vi "总磷氨氮公式读取.vi"(8 "error in (no error)":errorcluster caption="错误输入（无错误）", 9 "量程":enum16{"低量程", "高量程"}(ring), 10 "测量模式":enum16{"水样测量", "空白核查", "跨度核查", "标样核查", "加标回收"}(ring), 11 "测量参数":enum16{"氨氮", "总磷"}(ring)) -> (0 "error out":errorcluster caption="错误输出", 3 "公式":cluster{"X^2":dbl, "X":dbl, "b":dbl})   [LabVIEW 2016, in "氨氮.lvlib"]
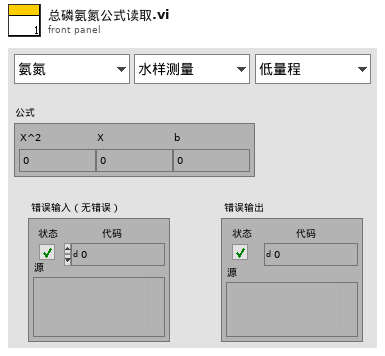
[diagram p1: front panel]
types:
  T1 = cluster{"FLOAT[0]":sgl, "FLOAT[1]":sgl, "FLOAT[2]":sgl}
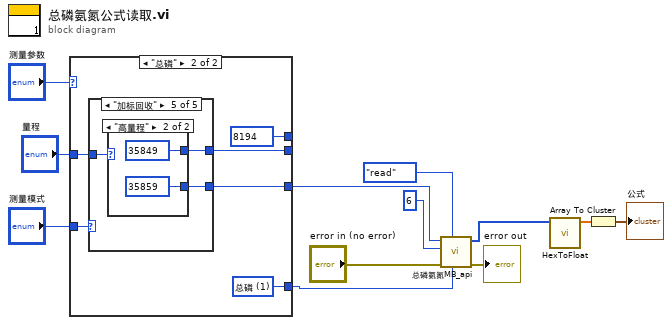
[diagram p0: block diagram]
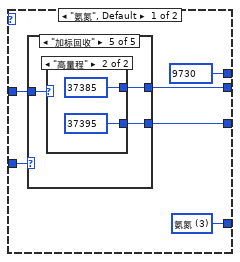
[diagram p2: hidden frame]
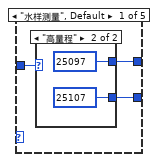
[diagram p3: hidden frame]
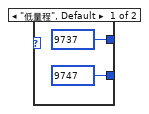
[diagram p4: hidden frame]
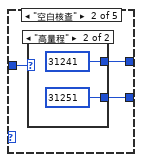
[diagram p5: hidden frame]
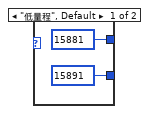
[diagram p6: hidden frame]
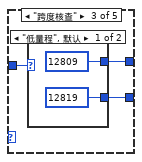
[diagram p7: hidden frame]
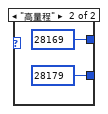
[diagram p8: hidden frame]
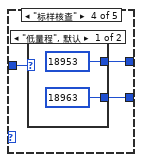
[diagram p9: hidden frame]
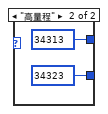
[diagram p10: hidden frame]
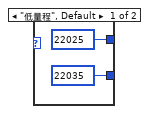
[diagram p11: hidden frame]
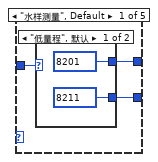
[diagram p12: hidden frame]
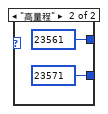
[diagram p13: hidden frame]
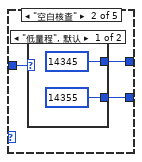
[diagram p14: hidden frame]
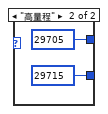
[diagram p15: hidden frame]
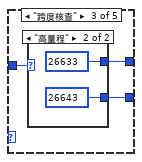
[diagram p16: hidden frame]
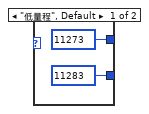
[diagram p17: hidden frame]
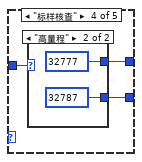
[diagram p18: hidden frame]
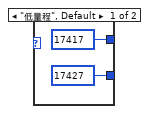
[diagram p19: hidden frame]
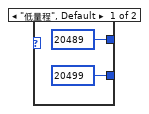
[diagram p20: hidden frame]
diagram:
  n1 = case shown="\"总磷\"" "测量参数" {
    tunnel: "测量模式" -> [w18 w59]
    tunnel: "量程" -> [w17 w58]
    tunnel: [w16 w57] -> w2
    tunnel: [w15 w56] -> w9
    tunnel: [w14 w55] -> _
    tunnel: [u16 9730 ("starting address") u16 8194 ("starting address")] -> _
    frame "氨氮", Default {
      w16 = u16 3 items=["总磷"=1, "氨氮"=3] ("站号")
      n2 = case shown="\"加标回收\"" w18 {
        tunnel: w17 -> [w21 w28 w35 w42 w49]
        tunnel: [w20 w27 w34 w41 w48] -> w15
        tunnel: [w19 w26 w33 w40 w47] -> w14
        frame "水样测量", Default {
          n3 = case shown="\"高量程\"" w21 {
            tunnel: [u16 9747 ("starting address") u16 25107 ("starting address")] -> w20
            tunnel: [u16 9737 ("starting address") u16 25097 ("starting address")] -> w19
            frame "低量程", Default {
            }
            frame "高量程" {
            }
          }
        }
        frame "空白核查" {
          n4 = case shown="\"高量程\"" w28 {
            tunnel: [u16 15891 ("starting address") u16 31251 ("starting address")] -> w27
            tunnel: [u16 15881 ("starting address") u16 31241 ("starting address")] -> w26
            frame "低量程", Default {
            }
            frame "高量程" {
            }
          }
        }
        frame "跨度核查" {
          n5 = case shown="\"低量程\", 默认" w35 {
            tunnel: [u16 12819 ("starting address") u16 28179 ("starting address")] -> w34
            tunnel: [u16 12809 ("starting address") u16 28169 ("starting address")] -> w33
            frame "低量程", Default {
            }
            frame "高量程" {
            }
          }
        }
        frame "标样核查" {
          n6 = case shown="\"低量程\", 默认" w42 {
            tunnel: [u16 18963 ("starting address") u16 34323 ("starting address")] -> w41
            tunnel: [u16 18953 ("starting address") u16 34313 ("starting address")] -> w40
            frame "低量程", Default {
            }
            frame "高量程" {
            }
          }
        }
        frame "加标回收" {
          n7 = case shown="\"高量程\"" w49 {
            tunnel: [u16 22035 ("starting address") u16 37395 ("starting address")] -> w48
            tunnel: [u16 22025 ("starting address") u16 37385 ("starting address")] -> w47
            frame "低量程", Default {
            }
            frame "高量程" {
            }
          }
        }
      }
    }
    frame "总磷" {
      w57 = u16 1 items=["总磷"=1, "氨氮"=3] ("站号")
      n8 = case shown="\"加标回收\"" w59 {
        tunnel: w58 -> [w62 w69 w76 w83 w90]
        tunnel: [w61 w68 w75 w82 w89] -> w56
        tunnel: [w60 w67 w74 w81 w88] -> w55
        frame "水样测量", Default {
          n9 = case shown="\"低量程\", 默认" w62 {
            tunnel: [u16 8211 ("starting address") u16 23571 ("starting address")] -> w61
            tunnel: [u16 8201 ("starting address") u16 23561 ("starting address")] -> w60
            frame "低量程", Default {
            }
            frame "高量程" {
            }
          }
        }
        frame "空白核查" {
          n10 = case shown="\"低量程\", 默认" w69 {
            tunnel: [u16 14355 ("starting address") u16 29715 ("starting address")] -> w68
            tunnel: [u16 14345 ("starting address") u16 29705 ("starting address")] -> w67
            frame "低量程", Default {
            }
            frame "高量程" {
            }
          }
        }
        frame "跨度核查" {
          n11 = case shown="\"高量程\"" w76 {
            tunnel: [u16 11283 ("starting address") u16 26643 ("starting address")] -> w75
            tunnel: [u16 11273 ("starting address") u16 26633 ("starting address")] -> w74
            frame "低量程", Default {
            }
            frame "高量程" {
            }
          }
        }
        frame "标样核查" {
          n12 = case shown="\"高量程\"" w83 {
            tunnel: [u16 17427 ("starting address") u16 32787 ("starting address")] -> w82
            tunnel: [u16 17417 ("starting address") u16 32777 ("starting address")] -> w81
            frame "低量程", Default {
            }
            frame "高量程" {
            }
          }
        }
        frame "加标回收" {
          n13 = case shown="\"高量程\"" w90 {
            tunnel: [u16 20499 ("starting address") u16 35859 ("starting address")] -> w89
            tunnel: [u16 20489 ("starting address") u16 35849 ("starting address")] -> w88
            frame "低量程", Default {
            }
            frame "高量程" {
            }
          }
        }
      }
    }
  }
  n14 = call "总磷氨氮MB_api.vi"("Slave ID"=w2, "STEP"=enum16{"open", "read", "write", "close"}."read", "Error in"="error in (no error)", "quantity"=u16 6, "starting address"=w9) -> ("error out"=→"error out":errorcluster, "Registers"=w7:u16[])  [unwired: 4 in, 1 out]
  n15 = call "HexToFloat.vi"("数组"=w7) -> ("FLOAT"=w6:sgl[])  [unwired: 10 in]
  n16 = Array To Cluster(array=w6) -> (cluster=→"公式":T1)
